vi "Global Strings.vi"() -> ()   [LabVIEW 2020, in "Output Sequencer.lvlib" / "Output Sequencer.lvclass"]
uses:
  Output Sequencer.lvclass
panel:
  in  "Unknown Variable Error (dialog)":string="Error in expression: \"%s\".\nUnknown variable \"%s\"."
  in  "Invalid Step Error":string="Step %d has an invalid step listed in action \"%s\". Make sure to select a valid step number between 0 and %d."
  in  "muParser Error":string="Error in expression: \"%s\". %s"
  in  "Unknown Variable Error":string="Error in expression: \"%s\". Unknown variable \"%s\"."
  in  "Unknown Channel Error":string="Error in expression: \"%s\". Unknown channel %s. Make sure to map referenced channels into the Output Sequencer plug-in by clicking the settings gear."
  in  "Analog Short":string="Analog %d"
  in  "Digital Short":string="Digital %d"
  in  "Reset sequence":string="Reset sequence"
  in  "State":string="State"
  in  "Execution State":string="Execution State"
  in  "Constants":string[](array[string])=["pi", "e", "true", "false"]
  in  "Functions":string[](array[string])=["sin", "cos", "tan", "asin", "acos", "atan", "sinh", "cosh", "tanh", "asinh", "acosh", "atanh", "log2", "log10", "log", "ln", "exp", "sqrt", "sign", "rint", "abs", "min", "max", "sum", "avg"]
  in  "Autocomplete Delimiters":string[](array[string])=[" ", "'", ";", "!", "=", ">", "<", "+", "-", "*", "/", "^", "(", ")", "%", "?", ":", "|", "&", "~"]
  in  "Disabled":string="Disabled"
  in  "Enabled":string="Enabled"
  in  "t":string="t"
  in  "False":string="False"
  in  "True":string="True"
  in  "Plug-in Version":string="1.0"
  in  "Analog Conditional Channels":string="Analog Conditional Channels"
  in  "Default":string="Default"
  in  "Digital Conditional Channels":string="Digital Conditional Channels"
  in  "Last":string="Last"
  in  "Analog Channel ID":string="A%d"
  in  "Digital Channel ID":string="D%d"
  in  "Total Cycles":string="Total Cycles"
  in  "Total Sequence Cycles":string="Total Sequence Cycles"
  in  "Time Left":string="Time Left"
  in  "Remaining Time in Step":string="Remaining Time in Current Step"
  in  "Step #":string="Step #"
  in  "Sequence Step":string="Sequence Step Number"
  in  "Internal Settings Message":string="Use \"Configure\" button to edit.\n\n<START>"
  in  "Internal Settings":string="Internal Settings. Use \"Configure\" button to edit."
  in  "Command":string="Configure"
  in  "Delimeter":string=";"
  in  "Digital Channel Name":string="Digital Channel %d"
  in  "Analog Channel Name":string="Analog Channel %d"
  in  "Default Mode Value":string="Wait for end of step"
  in  "Mode Enum Values":string[](array[string])=["Wait for end of step", "Repeat channel values"]
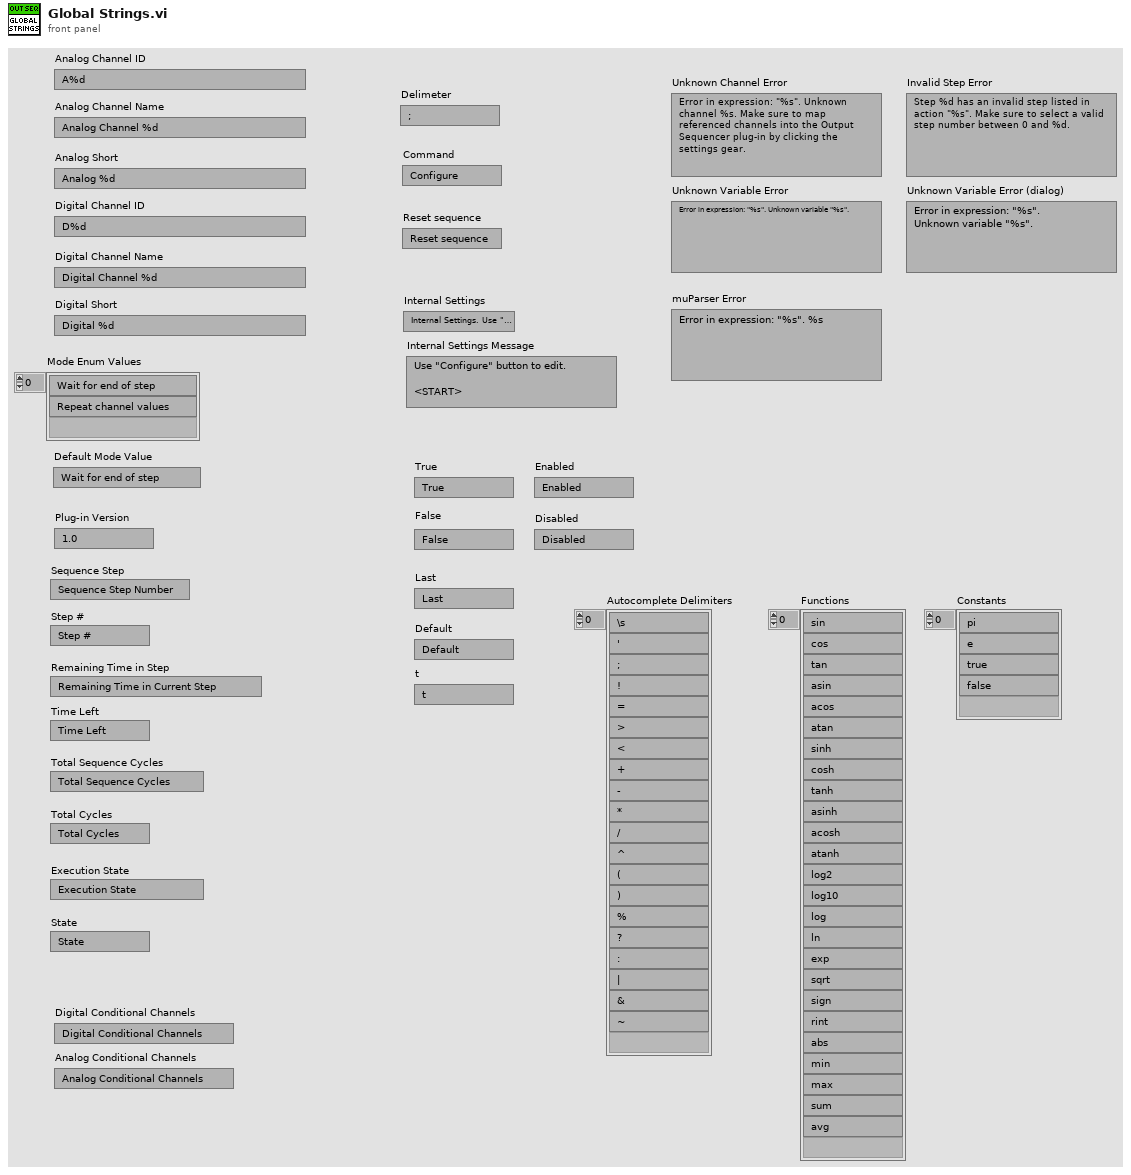
[diagram p1: front panel]
diagram:
